vi "Connect.vi"(8 "error in (no error)":errorcluster, 11 "3446X in":refnum<class "3446X.lvclass">) -> (0 "error out":errorcluster, 3 "3446X out":refnum<class "3446X.lvclass">)   [LabVIEW 2018, in "3446X.lvlib" / "3446X.lvclass"]
uses:
  3446X.lvclass
  3446X.lvclass/3446X.ctl
  <instrlib>/Agilent 3446X Series/Agilent 3446X Series.lvlib
  PPLs/DMM/Parent/DMM.lvlibp/DMM.lvclass
  C:/Projects/LabVIEW/PPLs/DMM/Parent/DMM.lvlibp/DMM.lvclass
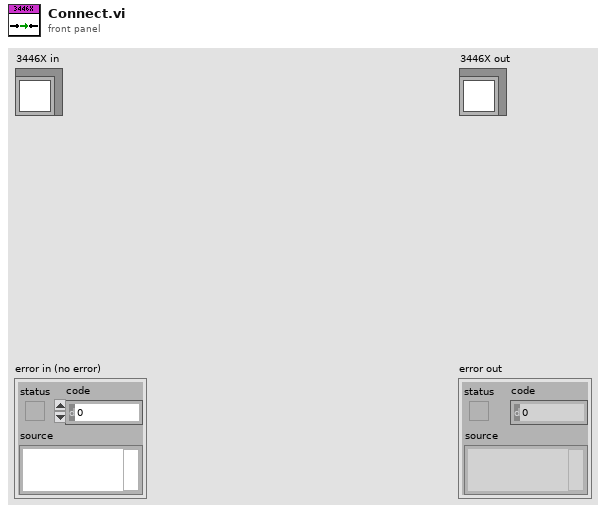
[diagram p1: front panel]
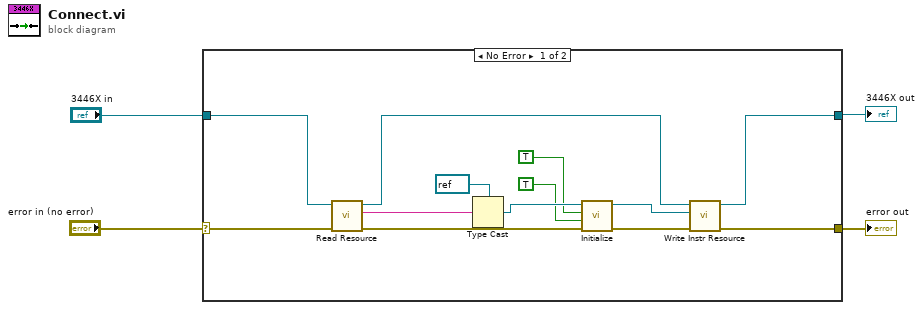
[diagram p0: block diagram]
diagram:
  n1 = case shown="No Error" "error in (no error)" {
    selector: "error in (no error)" -> [w17 w18]
    tunnel: "3446X in" -> [w16 w19]
    tunnel: [w9 w19] -> w2
    tunnel: [w10 w18] -> w1
    frame No Error {
      n2 = call "Read Resource.vi"("error in (no error)"=w17, "DMM in"=w16) -> ("error out"=w13:errorcluster, "Resource"=w15:string, "DMM out"=w12:refnum<class "3446X.lvclass">)  [unwired: 7 in]
      n3 = Type Cast(type=refnum<visa-resource-name> refnum ("VISA resource name"), x=w15) -> (*(type *) &x=w8:refnum<visa-resource-name>)
      n4 = call <instrlib>:"Initialize.vi"("error in (no error)"=w13, "Reset (True)"=TRUE, "ID Query (True)"=TRUE, "VISA resource name"=w8) -> ("error out"=w11:errorcluster, "VISA resource name out"=w7:refnum<visa-resource-name>)  [unwired: 6 in]
      n5 = call "Write Instr Resource.vi"("error in (no error)"=w11, "Instr Resource"=w7, "3446X in"=w12) -> ("error out"=w10:errorcluster, "3446X out"=w9:refnum<class "3446X.lvclass">)  [unwired: 7 in]
    }
    frame Error {
    }
  }
  "error out" <- w1
  "3446X out" <- w2
